vi "PPL RT Driver VI_InlineAsync.vi"(7 "Operation":T1, 11 "Device Reference in":T2 format="%.0x") -> (0 "Error Code":i32)   [LabVIEW 2020]
uses:
  <vilib>/NI/NIVS Inline Async API/_VS Inline Async API/VS Inline Async API/VS Inline Async API.lvclass
  <vilib>/NI VeriStand/Custom Device API/Custom Device API.lvlib
  <vilib>/NI VeriStand/Custom Device Tools/Custom Device Utility Library/Custom Device Utility Library.lvlib
  <vilib>/NI VeriStand/Custom Device API/Get Item Property (Variant).vi
  <vilib>/NI VeriStand/Custom Device API/Data Reference.ctl
  <vilib>/NI VeriStand/Custom Device API/Block Data Reference.ctl
  <vilib>/NI VeriStand/Custom Device API/Custom Device Item Ref.ctl
  <vilib>/NI VeriStand/Custom Device API/Hardware Interface Driver VI Operation.ctl
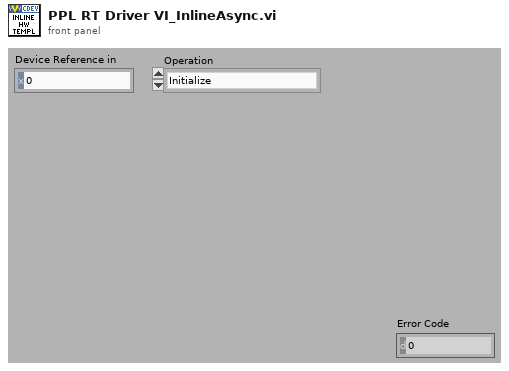
[diagram p1: front panel]
types:
  T1 = typedef "Custom Device API.lvlib/Hardware Interface Driver VI Operation.ctl" = enum16{"Initialize", "Start", "Read Data from HW", "Write Data to HW", "Close"}
  T2 = typedef "Custom Device API.lvlib/Custom Device Item Ref.ctl" = u64
  T3 = cluster{"Async":refnum<class "VS Inline Async API.lvclass">, "Settings":cluster{"Name":string, "Async Init Timeout":u16}}
  T4 = typedef "Custom Device API.lvlib/Block Data Reference.ctl" = cluster{"Data Reference":T5, "Offset":u64, "Length":u64}
  T5 = typedef "Custom Device API.lvlib/Data Reference.ctl" = i32
  T6 = cluster{"Name":string, "Async Init Timeout":u16, "Compiled.InlineAsync.Settings":cluster{"Read":cluster{"Refs":T4[], "Values":dbl[]}[], "Write":cluster{"Refs":T4[], "Values":dbl[]}[], "ReadWrite":cluster{"Refs":T5[], "Values":dbl[], "Reset Values":dbl[]}[], "LUT":variant}}
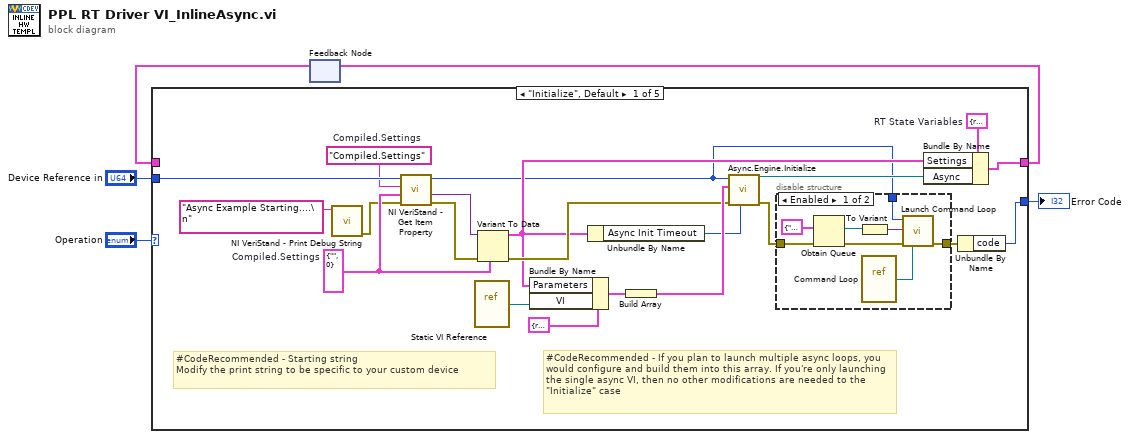
[diagram p0: block diagram]
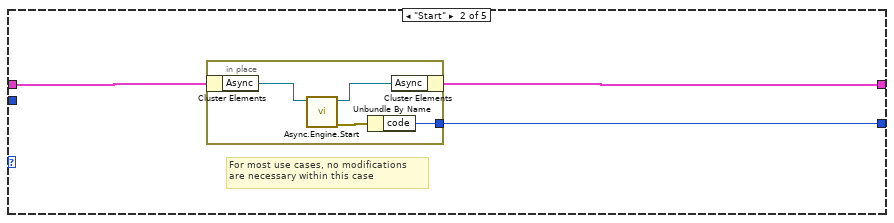
[diagram p3: hidden frame]
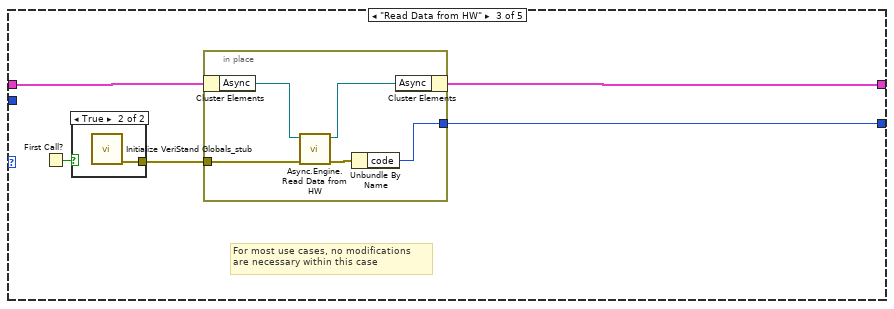
[diagram p4: hidden frame]
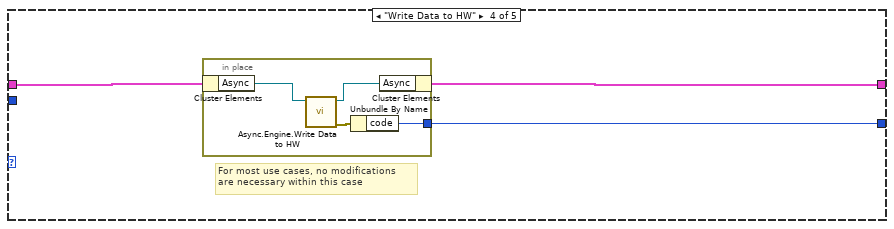
[diagram p6: hidden frame]
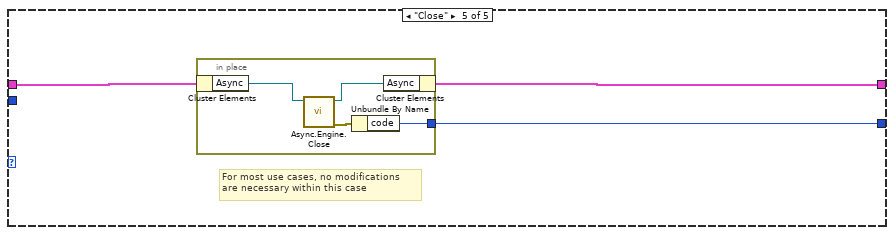
[diagram p7: hidden frame]
diagram:
  n1 = feedback #1() -> (w3:T3)  [unwired: 1 out]
  n2 = case shown="\"Initialize\", Default" "Operation" {
    tunnel: [w24 w37 w45 w54 w62] -> w4
    tunnel: w3 -> [_ w38 w47 w55 w63]
    tunnel: "Device Reference in" -> [w21 _ _ _ _]
    tunnel: [w26 w36 w46 w56 w61] -> w1
    frame "Initialize", Default {
      w16 = T3 {"Async"=refnum, "Settings"={"Name"="", "Async Init Timeout"=0}}  # RT State Variables
      w17 = cluster{"Name":string, "Async Init Timeout":u16} {"Name"="", "Async Init Timeout"=0}  # Compiled.Settings
      w18 = "Compiled.Settings"  # Compiled.Settings
      # "#CodeRecommended - Starting string\nModify the print string to be specific to your custom device"
      # "#CodeRecommended - If you plan to launch multiple async loops, you would configure and build them into this array. If you're only launching the single async VI, then no other modifications are needed to the \"Initialize\" case"
      n3 = call <vilib>:"NI VeriStand - Print Debug String.vi"("Message"="Async Example Starting....\n") -> ("error out"=w13:errorcluster)  [unwired: 10 in]
      n4 = call-poly <vilib>:"NI VeriStand - Get Item Property.vi"("error in (no error)"=w13, "Default Value"=w17, "Property Name"=w18, "Item Ref in"=w21) -> ("error out"=w20:errorcluster, "Value"=w19:variant, "Item Ref out"=w6:T2)  [unwired: 4 in, 1 out]
      n5 = vi-ref "Static VI Reference"() -> ("vi reference"=w11:refnum<vi>)
      n6 = Variant To Data(error in=w20, type=w17, Variant=w19) -> (data=w10:cluster{"Name":string, "Async Init Timeout":u16}, error out=w14:errorcluster)
      n7 = Bundle By Name(cluster=cluster{"VI":refnum<vi>, "Parameters":variant} {"VI"=refnum, "Parameters"=variant} ("Process"), "Parameters"=w10, "VI"=w11) -> (w22:cluster{"VI":refnum<vi>, "Parameters":variant})
      n8 = Unbundle By Name(w10) -> ("Async Init Timeout"=w9:u16)
      n9 = Build Array(w22) -> (w15:cluster{"VI":refnum<vi>, "Parameters":variant}[])
      n10 = call <vilib>:"Async.Engine.Initialize.vi"("Timeout (ms) (5000)"=w9, "error in (no error)"=w14, "Processes"=w15, "Custom Device Ref"=w6) -> ("error out"=w8:errorcluster, "Async"=w25:refnum<class "VS Inline Async API.lvclass">)  [unwired: 6 in]
      n11 = disable-structure shown="Enabled" {
        disable-tunnel: w8 -> [w30 w35]
        disable-tunnel: [w31 w35] -> w7
        disable-tunnel: w6 -> [w27 _]
        frame Enabled {
          n12 = Obtain Queue(element data type=T6 {"Name"="", "Async Init Timeout"=0, "Compiled.InlineAsync.Settings"={"Read"=[], "Write"=[], "ReadWrite"=[], "LUT"=variant}} ("Reconfigure.Settings.ctl"), error in (no error)=w30) -> (queue out=w34:refnum<queue>, error out=w32:errorcluster)  [unwired: 3 in, 1 out]
          n13 = To Variant(anything=w34) -> (Variant=w33:variant)
          n14 = vi-ref "Command Loop.vi"() -> (w29:refnum<vi>)
          n15 = call "Launch Command Loop.vi"("VI Refnum"=w29, "error in"=w32, "Queue Refs"=w33, "Device Reference in"=w27) -> ("error out"=w31:errorcluster)  [unwired: 7 in]
        }
        frame Disabled {
        }
      }
      n16 = Bundle By Name(cluster=w16, "Settings"=w10, "Async"=w25) -> (w24:T3)
      n17 = Unbundle By Name(w7) -> ("code"=w26:i32)
    }
    frame "Start" {
      # "For most use cases, no modifications \nare necessary within this case"
      n18 = in-place {
        in-place-border: [w39] -> w36
        n19 = in-place-cluster #2(w38) -> ("Async"=w42:refnum<class "VS Inline Async API.lvclass">)
        n20 = call <vilib>:"Async.Engine.Start.vi"("VS Inline Async API in"=w42) -> ("error out"=w40:errorcluster, "VS Inline Async API out"=w41:refnum<class "VS Inline Async API.lvclass">)  [unwired: 9 in]
        n21 = Unbundle By Name(w40) -> ("code"=w39:i32)
        n22 = in-place-cluster #2("Async"=w41) -> (w37:T3)
      }
    }
    frame "Read Data from HW" {
      # "For most use cases, no modifications \nare necessary within this case"
      n23 = First Call?() -> (First Call?: T/F=w43:bool)
      n24 = case shown="True" w43 {
        tunnel: [_ w48] -> w44
        frame False {
        }
        frame True {
          n25 = call "Initialize VeriStand Globals_stub.vi"() -> ("error out"=w48:errorcluster)  [unwired: 11 in]
        }
      }
      n26 = in-place {
        in-place-border: [w51] -> w46
        in-place-border: w44 -> [w49]
        n27 = in-place-cluster #3(w47) -> ("Async"=w53:refnum<class "VS Inline Async API.lvclass">)
        n28 = call <vilib>:"Async.Engine.Read Data from HW.vi"("error in"=w49, "Async in"=w53) -> ("error out"=w50:errorcluster, "Async out"=w52:refnum<class "VS Inline Async API.lvclass">)  [unwired: 8 in]
        n29 = Unbundle By Name(w50) -> ("code"=w51:i32)
        n30 = in-place-cluster #3("Async"=w52) -> (w45:T3)
      }
    }
    frame "Write Data to HW" {
      # "For most use cases, no modifications \nare necessary within this case"
      n31 = in-place {
        in-place-border: [w60] -> w56
        n32 = in-place-cluster #4(w55) -> ("Async"=w58:refnum<class "VS Inline Async API.lvclass">)
        n33 = call <vilib>:"Async.Engine.Write Data to HW.vi"("VS Inline Async API in"=w58) -> ("error out"=w59:errorcluster, "VS Inline Async API out"=w57:refnum<class "VS Inline Async API.lvclass">)  [unwired: 9 in]
        n34 = Unbundle By Name(w59) -> ("code"=w60:i32)
        n35 = in-place-cluster #4("Async"=w57) -> (w54:T3)
      }
    }
    frame "Close" {
      # "For most use cases, no modifications \nare necessary within this case"
      n36 = in-place {
        in-place-border: [w65] -> w61
        n37 = in-place-cluster #5(w63) -> ("Async"=w67:refnum<class "VS Inline Async API.lvclass">)
        n38 = call <vilib>:"Async.Engine.Close.vi"("Async in"=w67) -> ("error out"=w64:errorcluster, "Async out"=w66:refnum<class "VS Inline Async API.lvclass">)  [unwired: 9 in]
        n39 = Unbundle By Name(w64) -> ("code"=w65:i32)
        n40 = in-place-cluster #5("Async"=w66) -> (w62:T3)
      }
    }
  }
  "Error Code" <- w1
  n41 = feedback-in #1(w4) -> ()
